vi "forceDemand.vi"(8 "error in (no error)":errorcluster, 9 "Force Demand":T1 format="%.1f", 10 "model":refnum<class "Model.lvclass">, 11 "InteractiveMotionState in":refnum<class "InteractiveMotionState.lvclass">) -> (0 "error out":errorcluster, 2 "model 2":refnum<class "Model.lvclass">, 3 "InteractiveMotionState out":refnum<class "InteractiveMotionState.lvclass">)   [LabVIEW 2013, in "InteractiveMotionState.lvclass"]
uses:
  InteractiveMotionState.lvclass
  Model/Model/Model.lvclass
  Typedefs/ForceDemand.ctl
  Typedefs/M2AADTTypedefs.lvlib
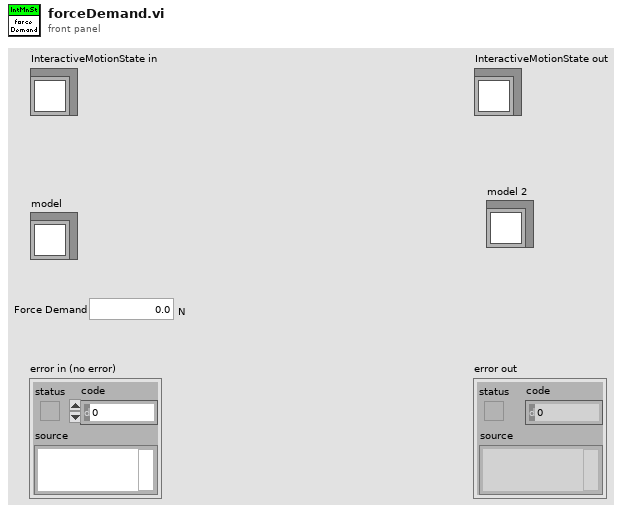
[diagram p1: front panel]
types:
  T1 = typedef "M2AADTTypedefs.lvlib/ForceDemand.ctl" = dbl[unit]
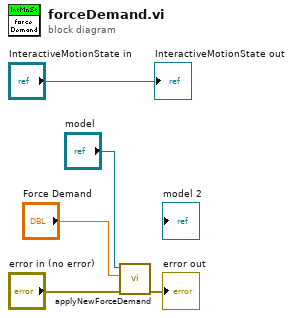
[diagram p0: block diagram]
diagram:
  n1 = call "applyNewForceDemand.vi"("error in (no error)"="error in (no error)", "Force Demand"="Force Demand", "Model in"="model") -> ("error out"=→"error out":errorcluster)  [unwired: 7 in, 1 out]
  "InteractiveMotionState out" <- "InteractiveMotionState in"
